vi "Document Property Node.vi"   [LabVIEW 2017, in "LabVIEW NPOI.lvlib" / "Document.lvclass"]
uses:
  Document.lvclass
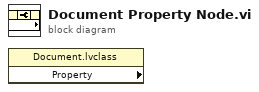
[diagram p0: block diagram]
diagram:
  n1 = property class="Document.lvclass" props=[]() -> ()  [unwired: 2 in, 3 out]
